vi "ziExample-AUXIn.vi"() -> ()   [LabVIEW 2009]
doc: "Control a Zurich instrument device via the LabOne Labview API. \nRequirements: Zurich Instruments MFLI, HF2 or UHFLI \nThis vi controls the aux outputs and reads the aux inputs.\n\n© Zurich Instruments AG, www.zhinst.com"
uses:
  <instrlib>/Zurich Instruments LabOne/Public/Data/ziTypeAuxInSample.ctl
  <instrlib>/Zurich Instruments LabOne/Public/Utility/ziTicksToS_vector.vi
  <instrlib>/Zurich Instruments LabOne/Public/Data/ziGetEventAuxInSample.vi
  <instrlib>/Zurich Instruments LabOne/Zurich Instruments LabOne.lvlib
panel:
  out "Error Out":errorcluster
  in  "Address":string="DEV"
  out "Selected Device":string
  in  "ramp":bool caption="Ramp Aux Out"
  in  "Samples":u32=1000
  out "Progress":dbl(slide) scale=0.0..1.0
  in  "run":bool
  in  "stop":bool
  out "Waveform":cluster{dbl[], "Val Ch0 (V)":dbl[]}[](graph)
  # "Tested Instruments:\n- MFLI\n- HF2LI\n- UHFLI"
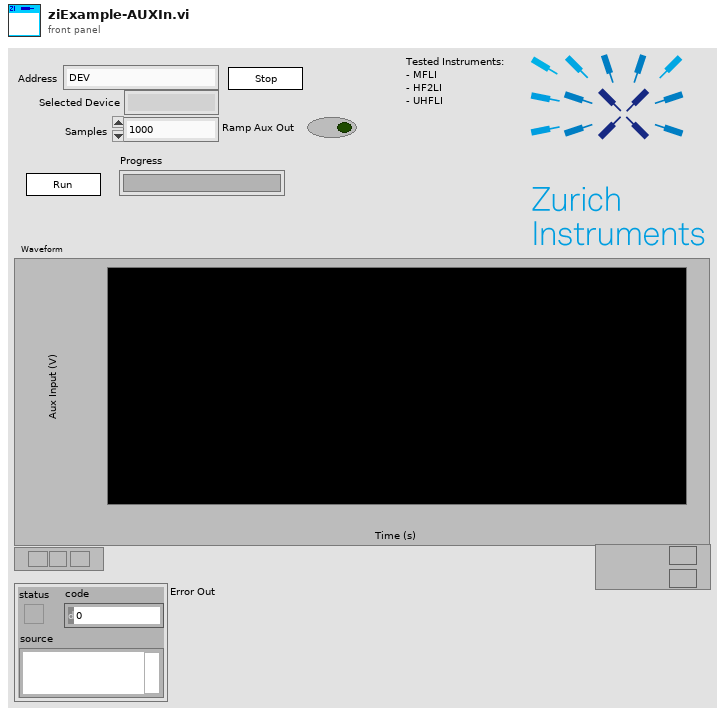
[diagram p1: front panel]
types:
  T1 = typedef "Zurich Instruments LabOne.lvlib/ziTypeHandle.ctl" = cluster{"handleValid":bool, "Conn":u64, "Path Prefix":string, "Handle":u64, "Connected":bool, "Clockbase(s)":dbl}
  T2 = typedef "Zurich Instruments LabOne.lvlib/ziTypeAuxInSample.ctl" = cluster{"Timestamp (ticks)":u64[], "Val Ch0 (V)":dbl[], "Val Ch1 (V)":dbl[]}
  T3 = typedef "Zurich Instruments LabOne.lvlib/ziTypePollType.ctl" = enum16{"NONE", "DOUBLE_DATA", "INTEGER_DATA", "DEMOD_SAMPLE", "SCOPE_WAVE_HF2", "AUXIN_SAMPLE", "DIO_SAMPLE", "BYTE_ARRAY", "PWA_WAVE", "9", "10", "11", "12", "13", "14", "15", "TREE_CHANGE_DEPRI", "17", "ERROR", "19", "20", "21", "22", "23", "24", "25", "26", "27", "28", "29", "30", "31", "DOUBLE_DATA_TS", "INTEGER_DATA_TS", "34", "SCOPE_WAVE", "SCOPE_WAVE_EX", "37", "BYTE_ARRAY_TS", "39", "40", "41", "42", "43", "44", "45", "CNT_DATA", "47", "TREE_CHANGE", "49", "50", "51", "52", "53", "54", "55", "56", "57", "58", "59", "60", "61", "62", "63", "SWEEPER_DATA", "SPECTRUM_DATA", "ADVISOR_DATA", "VECTOR_DATA", "IMP_DATA"}
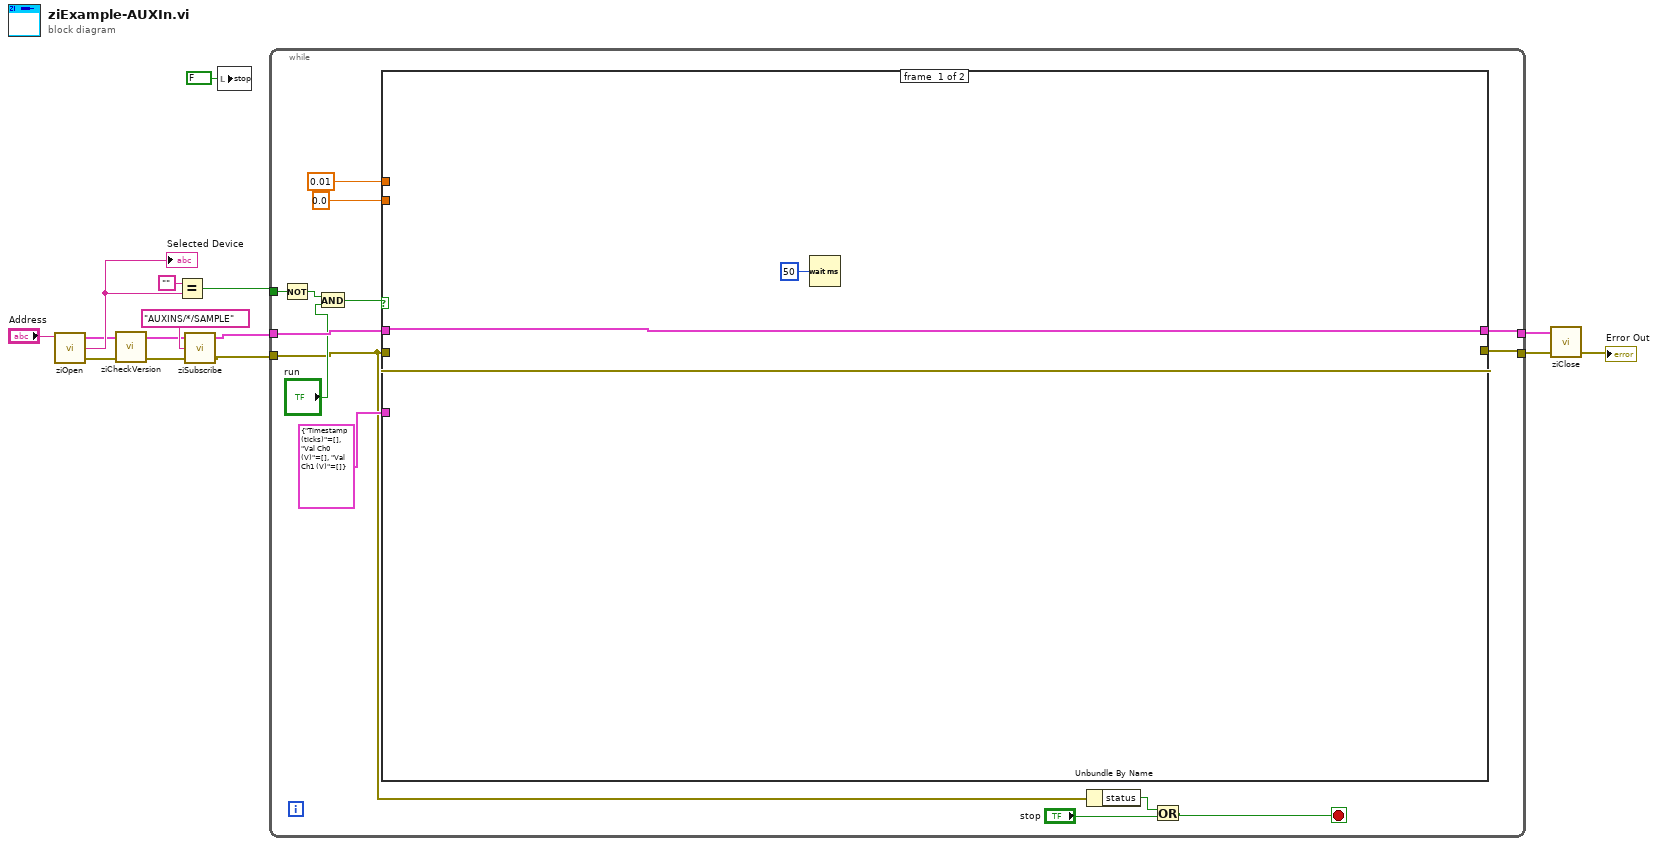
[diagram p0: block diagram]
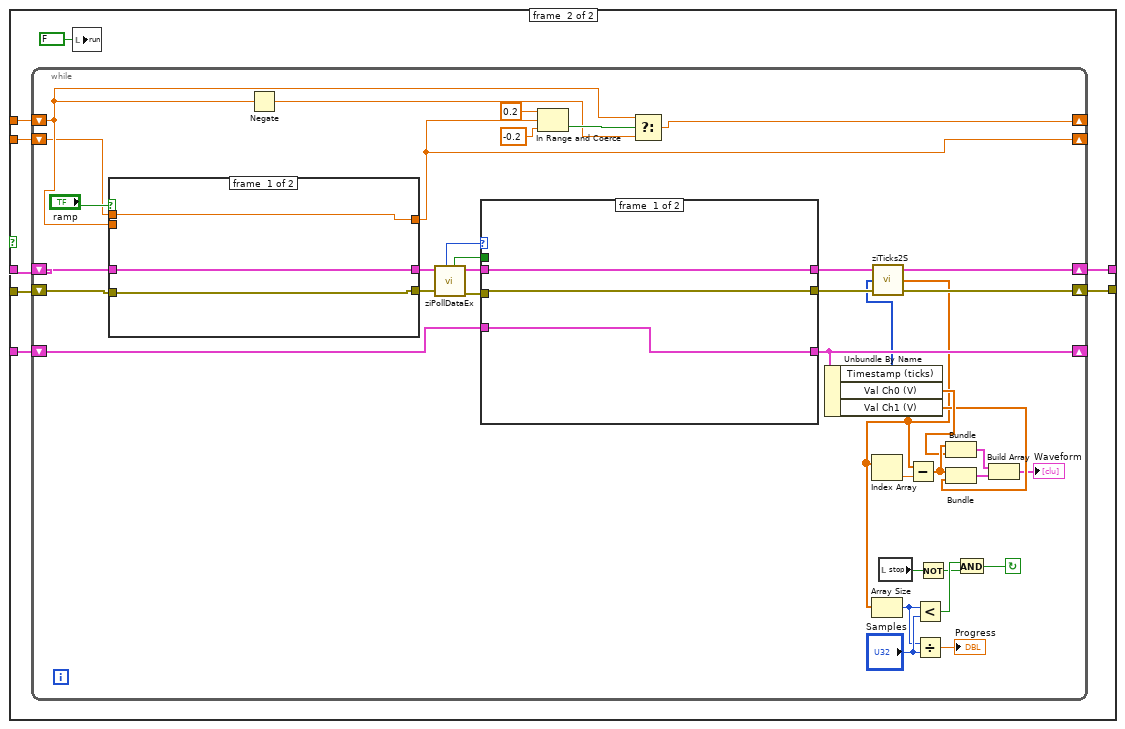
[diagram p2: hidden frame]
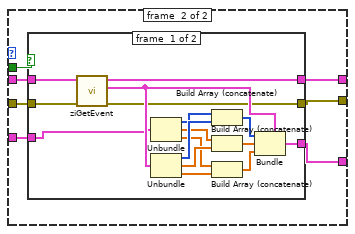
[diagram p3: hidden frame]
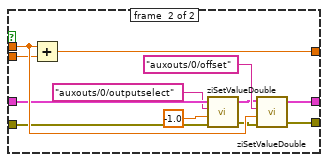
[diagram p5: hidden frame]
diagram:
  n1 = call <instrlib>:"ziOpen.vi"("Address"="Address") -> ("Error Out"=w3:errorcluster, "Selected Device"=w11:string, "HandleOut"=w4:T1)  [unwired: 1 in, 2 out]
  "Selected Device" <- w11
  n2 = call <instrlib>:"ziCheckVersion.vi"("Handle In"=w4, "Error In"=w3) -> ("Handle Out"=w1:T1, "Error Out"=w2:errorcluster)  [unwired: 11 in, 1 out]
  n3 = Equal?(x="", y=w11) -> (x = y?=w5:bool)
  n4 = call <instrlib>:"ziSubscribe.vi"("error in"=w2, "Path ()"="AUXINS/*/SAMPLE", "Handle In"=w1) -> ("error out"=w6:errorcluster, "Handle Out"=w7:T1)  [unwired: 1 out]
  n5 = local write "stop"(FALSE ("run")) -> ()
  n6 = while {
    tunnel: [w29] -> w13
    tunnel: [w28] -> w12
    tunnel: w7 -> [w27]
    tunnel: w6 -> [w16]
    tunnel: w5 -> [w25]
    stop <- w17 stop-if-true
    n7 = Not(x=w25) -> (.not. x?=w26:bool)
    n8 = And(x=w26, y="run") -> (x .and. y?=w23:bool)
    n9 = case shown="True" w23 {
      tunnel: [w31 w39] -> w29
      tunnel: [w30 w38] -> w28
      tunnel: w27 -> [w30 w37]
      tunnel: w16 -> [w31 w36]
      tunnel: T2 {"Timestamp (ticks)"=[], "Val Ch0 (V)"=[], "Val Ch1 (V)"=[]} ("AuxIn Out") -> [_ w35]
      tunnel: 0.01 -> [_ w34]
      tunnel: 0.0 -> [_ w33]
      frame #0 {
        n10 = Wait (ms)(milliseconds to wait=50) -> ()  [unwired: 1 out]
      }
      frame #1 {
        n11 = while {
          shift-right: [w53] -> w38
          shift-left: w37 -> [w76]
          shift-right: [w54] -> w39
          shift-left: w36 -> [w77]
          shift-right: [w57] -> _
          shift-left: w35 -> [w58]
          shift-right: [w44] -> _
          shift-left: w34 -> [w43]
          shift-right: [w41] -> _
          shift-left: w33 -> [w42]
          stop <- w68 continue-if-true
          n12 = case shown="True" "ramp" {
            tunnel: w77 -> [w110 w117]
            tunnel: w76 -> [w109 w118]
            tunnel: w42 -> [w111 w122]
            tunnel: w43 -> [_ w112]
            tunnel: [w111 w121] -> w41
            tunnel: [w110 w120] -> w75
            tunnel: [w109 w119] -> w74
            frame #0 {
            }
            frame #1 {
              n13 = Add(x=w122, y=w112) -> (x+y=w121:dbl)
              n14 = call <instrlib>:"ziSetValueDouble.vi"("Error In"=w117, "Value"=-1.0, "Path"="auxouts/0/outputselect", "Handle In"=w118) -> ("Error Out"=w116:errorcluster, "Handle Out"=w115:T1)  [unwired: 1 out]
              n15 = call <instrlib>:"ziSetValueDouble.vi"("Error In"=w116, "Value"=w122, "Path"="auxouts/0/offset", "Handle In"=w115) -> ("Error Out"=w120:errorcluster, "Handle Out"=w119:T1)  [unwired: 1 out]
            }
          }
          n16 = Negate(x=w43) -> (-x=w61:dbl)
          n17 = call <instrlib>:"ziPollDataEx.vi"("error in"=w75, "Handle In"=w74) -> ("error out"=w69:errorcluster, "Handle Out"=w70:T1, "Timed Out"=w79:bool, "ziValueType"=w65:T3)  [unwired: 2 in, 4 out]
          n18 = case shown="\"AUXIN_SAMPLE\"" w65 {
            tunnel: w79 -> [_ w89]
            tunnel: w70 -> [w82 w88]
            tunnel: [w82 w87] -> w56
            tunnel: w69 -> [w81 w86]
            tunnel: [w81 w85] -> w55
            tunnel: [w80 w84] -> w57
            tunnel: w58 -> [w80 w83]
            frame #0 {
            }
            frame #1 {
              n19 = case shown="False" w89 {
                tunnel: w88 -> [w105 w108]
                tunnel: [w96 w108] -> w87
                tunnel: w86 -> [w104 w107]
                tunnel: [w97 w107] -> w85
                tunnel: [w94 w106] -> w84
                tunnel: w83 -> [w93 w106]
                frame #0 {
                  n20 = call-poly <instrlib>:"ziGetEvent.vi"("Error In"=w104, "Handle In"=w105) -> ("Error Out"=w97:errorcluster, "AuxIn Out"=w101:T2, "Handle Out"=w96:T1)  [unwired: 7 in]
                  n21 = Unbundle(w93) -> ("Timestamp (ticks)"=w90:u64[], "Val Ch0 (V)"=w92:dbl[], "Val Ch1 (V)"=w91:dbl[])
                  n22 = Unbundle(w101) -> ("Timestamp (ticks)"=w95:u64[], "Val Ch0 (V)"=w102:dbl[], "Val Ch1 (V)"=w103:dbl[])
                  n23 = Build Array (concatenate)(w90, w95) -> (w100:u64[])
                  n24 = Build Array (concatenate)(w92, w102) -> (w99:dbl[])
                  n25 = Build Array (concatenate)(w91, w103) -> (w98:dbl[])
                  n26 = Bundle(cluster=w101, "Timestamp (ticks)"=w100, "Val Ch0 (V)"=w99, "Val Ch1 (V)"=w98) -> (w94:T2)
                }
                frame #1 {
                }
              }
            }
          }
          n27 = In Range and Coerce(upper limit=0.2 ("y"), x=w41, lower limit=-0.2 ("y")) -> (In Range?=w62:bool)  [unwired: 1 out]
          n28 = Select(t=w43, s=w62, f=w61) -> (s? t:f=w44:dbl)
          n29 = Unbundle By Name(w57) -> ("Timestamp (ticks)"=w52:u64[], "Val Ch0 (V)"=w51:dbl[], "Val Ch1 (V)"=w50:dbl[])
          n30 = call-poly <instrlib>:"ziTicks2S.vi"("Error In"=w55, "Timestamp (ticks)"=w52, "Handle In"=w56) -> ("Error Out"=w54:errorcluster, "Timestamp(s)"=w47:dbl[], "Handle Out"=w53:T1)
          n31 = Index Array(array=w47) -> (element=w48:dbl)  [unwired: 1 in]
          n32 = Array Size(array=w47) -> (size(s)=w72:i32)
          n33 = local read "stop"() -> (w67:bool)
          n34 = Subtract(x=w47, y=w48) -> (x-y=w60:dbl[])
          n35 = Less?(x=w72, y="Samples") -> (x < y?=w78:bool)
          n36 = Divide(x=w72, y="Samples") -> (x/y=→"Progress":dbl)
          n37 = Not(x=w67) -> (.not. x?=w66:bool)
          n38 = Bundle(w60, "Val Ch0 (V)"=w51) -> (w59:cluster{dbl[], "Val Ch0 (V)":dbl[]})  [unwired: 1 out]
          n39 = Bundle(w60, "Val Ch1 (V)"=w50) -> (w49:cluster{dbl[], "Val Ch1 (V)":dbl[]})  [unwired: 1 out]
          n40 = And(x=w78, y=w66) -> (x .and. y?=w68:bool)
          n41 = Build Array(w59, w49) -> (→"Waveform":cluster{dbl[], "Val Ch1 (V)":dbl[]}[])
        }
        n42 = local write "run"(FALSE ("run")) -> ()
      }
    }
    n43 = Unbundle By Name(w16) -> ("status"=w19:bool)
    n44 = Or(x=w19, y="stop") -> (x .or. y?=w17:bool)
  }
  n45 = call <instrlib>:"ziClose.vi"("Error In"=w13, "Handle In"=w12) -> ("Error Out"=→"Error Out":errorcluster)  [unwired: 3 out]
